vi "Maxi Gauge-ConvertEngEngInt.vi"(7 "W/R [W: Int in; Str out ]":bool, 8 "Integer1 in":u8 max=5, 9 "Eng2 in":dbl format="%.2e", 10 "Eng1 in":dbl format="%.2e", 11 "String in":string) -> (0 "Integer1 out":u8 max=5, 1 "Eng2 out":dbl format="%.2e", 2 "Eng1 out":dbl format="%.2e", 3 "String out":string)   [LabVIEW 2012, in "Maxi Gauge.lvlib"]
uses:
  Maxi Gauge.lvlib
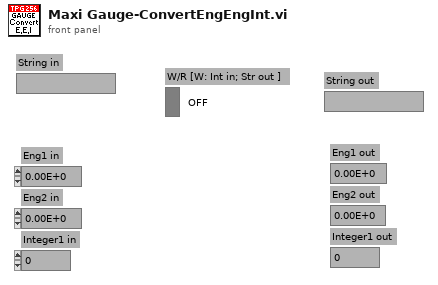
[diagram p1: front panel]
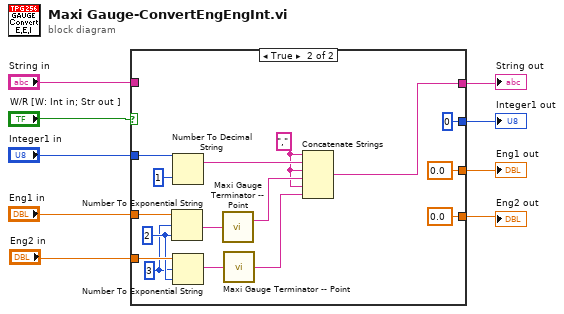
[diagram p0: block diagram]
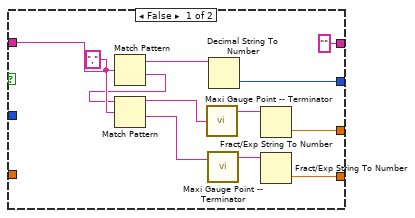
[diagram p2: hidden frame]
diagram:
  n1 = case shown="True" "W/R [W: Int in; Str out ]" {
    tunnel: "Integer1 in" -> [_ w37]
    tunnel: "Eng1 in" -> [_ w36]
    tunnel: "Eng2 in" -> [_ w35]
    tunnel: ["" w29] -> w5
    tunnel: "String in" -> [w18 _]
    tunnel: [w17 0] -> w3
    tunnel: [w12 0.0] -> w2
    tunnel: [w11 0.0] -> w1
    frame False {
      w20 = "," ("regular expression")
      n2 = Match Pattern(string=w18, regular expression=w20) -> (before substring=w21:string, after substring=w19:string)  [unwired: 1 in, 2 out]
      n3 = Match Pattern(string=w19, regular expression=w20) -> (before substring=w16:string, after substring=w15:string)  [unwired: 1 in, 2 out]
      n4 = call "Maxi Gauge Point -- Terminator.vi"("Eingangstring"=w16) -> ("Ausgangstring"=w14:string)
      n5 = call "Maxi Gauge Point -- Terminator.vi"("Eingangstring"=w15) -> ("Ausgangstring"=w13:string)
      n6 = Decimal String To Number(string=w21) -> (number=w17:i32)  [unwired: 2 in, 1 out]
      n7 = Fract/Exp String To Number(string=w14) -> (number=w11:dbl)  [unwired: 3 in, 1 out]
      n8 = Fract/Exp String To Number(string=w13) -> (number=w12:dbl)  [unwired: 3 in, 1 out]
    }
    frame True {
      w22 = i16 3 ("width (-)")
      w23 = i16 2 ("width (-)")
      w25 = ","
      n9 = Number To Exponential String(number=w36, precision (6)=w23, 3:w22) -> (E-format string=w34:string)  [unwired: 1 in]
      n10 = Number To Decimal String(number=w37, width (-)=i16 1) -> (decimal integer string=w32:string)
      n11 = Number To Exponential String(number=w35, precision (6)=w23, 3:w22) -> (E-format string=w33:string)  [unwired: 1 in]
      n12 = call "Maxi Gauge Terminator -- Point.vi"("Eingangstring"=w34) -> ("Ausgangstring"=w31:string)
      n13 = call "Maxi Gauge Terminator -- Point.vi"("Eingangstring"=w33) -> ("Ausgangstring"=w30:string)
      n14 = Concatenate Strings(w25, w32, w25, w31, w25, w30) -> (w29:string)
    }
  }
  "String out" <- w5
  "Integer1 out" <- w3
  "Eng1 out" <- w1
  "Eng2 out" <- w2
